vi "SQL_删除所有行.vi"(8 "error in (no error)":errorcluster, 10 "表名":string="DELETE FROM table_name", 11 "connection reference":T1) -> (0 "error out":errorcluster)   [LabVIEW 2014]
uses:
  <vilib>/addons/database/Connection.llb/Conn ObjectReference.ctl
  <vilib>/addons/database/Connection.llb/Conn Execute.vi
  <vilib>/addons/database/Recordset.llb/Rec Destroy - Connection.vi
  <vilib>/addons/database/NI_Database_API.lvlib
panel:
  # "语法："
  # "UPDATE 表名称 SET 列名称 = 新值 WHERE 列名称 = 某值"
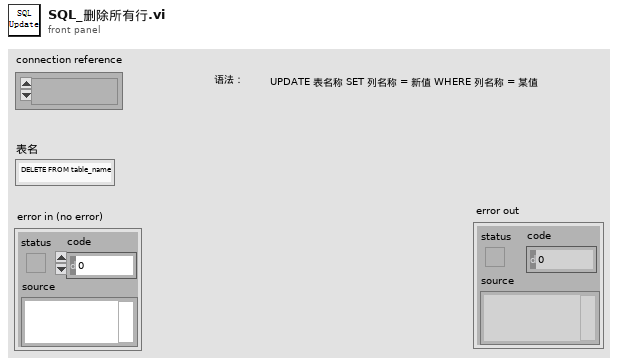
[diagram p1: front panel]
types:
  T1 = typedef "NI_Database_API.lvlib/Conn ObjectReference.ctl" = refnum<k1>
  T2 = typedef "NI_Database_API.lvlib/Rec ObjectReference.ctl" = refnum<k1>
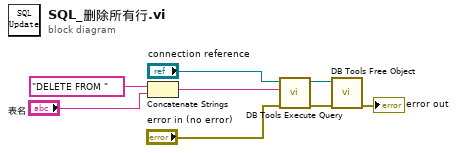
[diagram p0: block diagram]
diagram:
  n1 = Concatenate Strings("DELETE FROM ", "表名") -> (w1:string)
  n2 = call-poly <vilib>:"DB Tools Execute Query.vi"("error in (no error)"="error in (no error)", "SQL query"=w1, "connection reference"="connection reference") -> ("error out"=w4:errorcluster, "recordset reference"=w5:T2)  [unwired: 5 in]
  n3 = call-poly <vilib>:"DB Tools Free Object.vi"("error in (no error)"=w4, "recordset reference"=w5) -> ("error out"=→"error out":errorcluster)  [unwired: 8 in, 1 out]
